vi "2022_day12.vi"() -> ()   [LabVIEW 2021]
uses:
  <vilib>/Utility/miscctls.llb/LVRowAndColumnTypeDef.ctl
panel:
  out "Table Control":string[][](table)
  out "Array":string[][](array[string])
  out "Searching progress":i32[][](array[numeric])
  out "Input Data":i32[][](array[numeric])
  out "Task 1":i32
  in  "Switch":bool caption="Ex. Data  vs.  User Data"
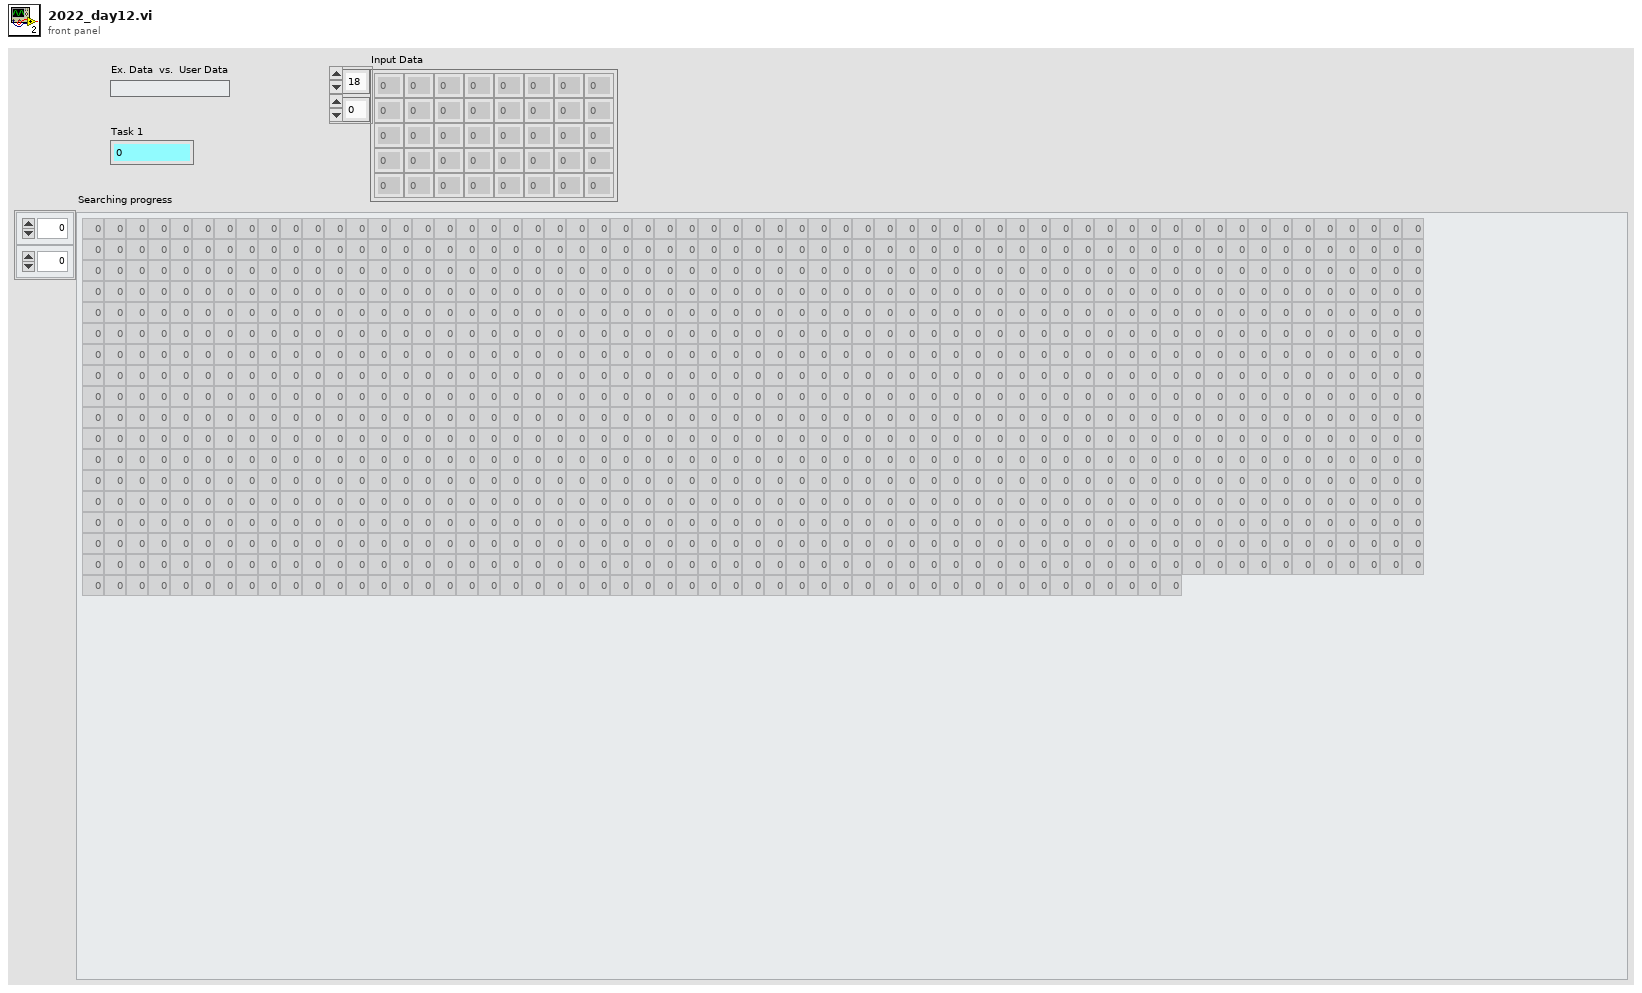
[diagram p1: front panel]
types:
  T1 = typedef "LVRowAndColumnTypeDef.ctl" = cluster{"Row":i32, "Column":i32}
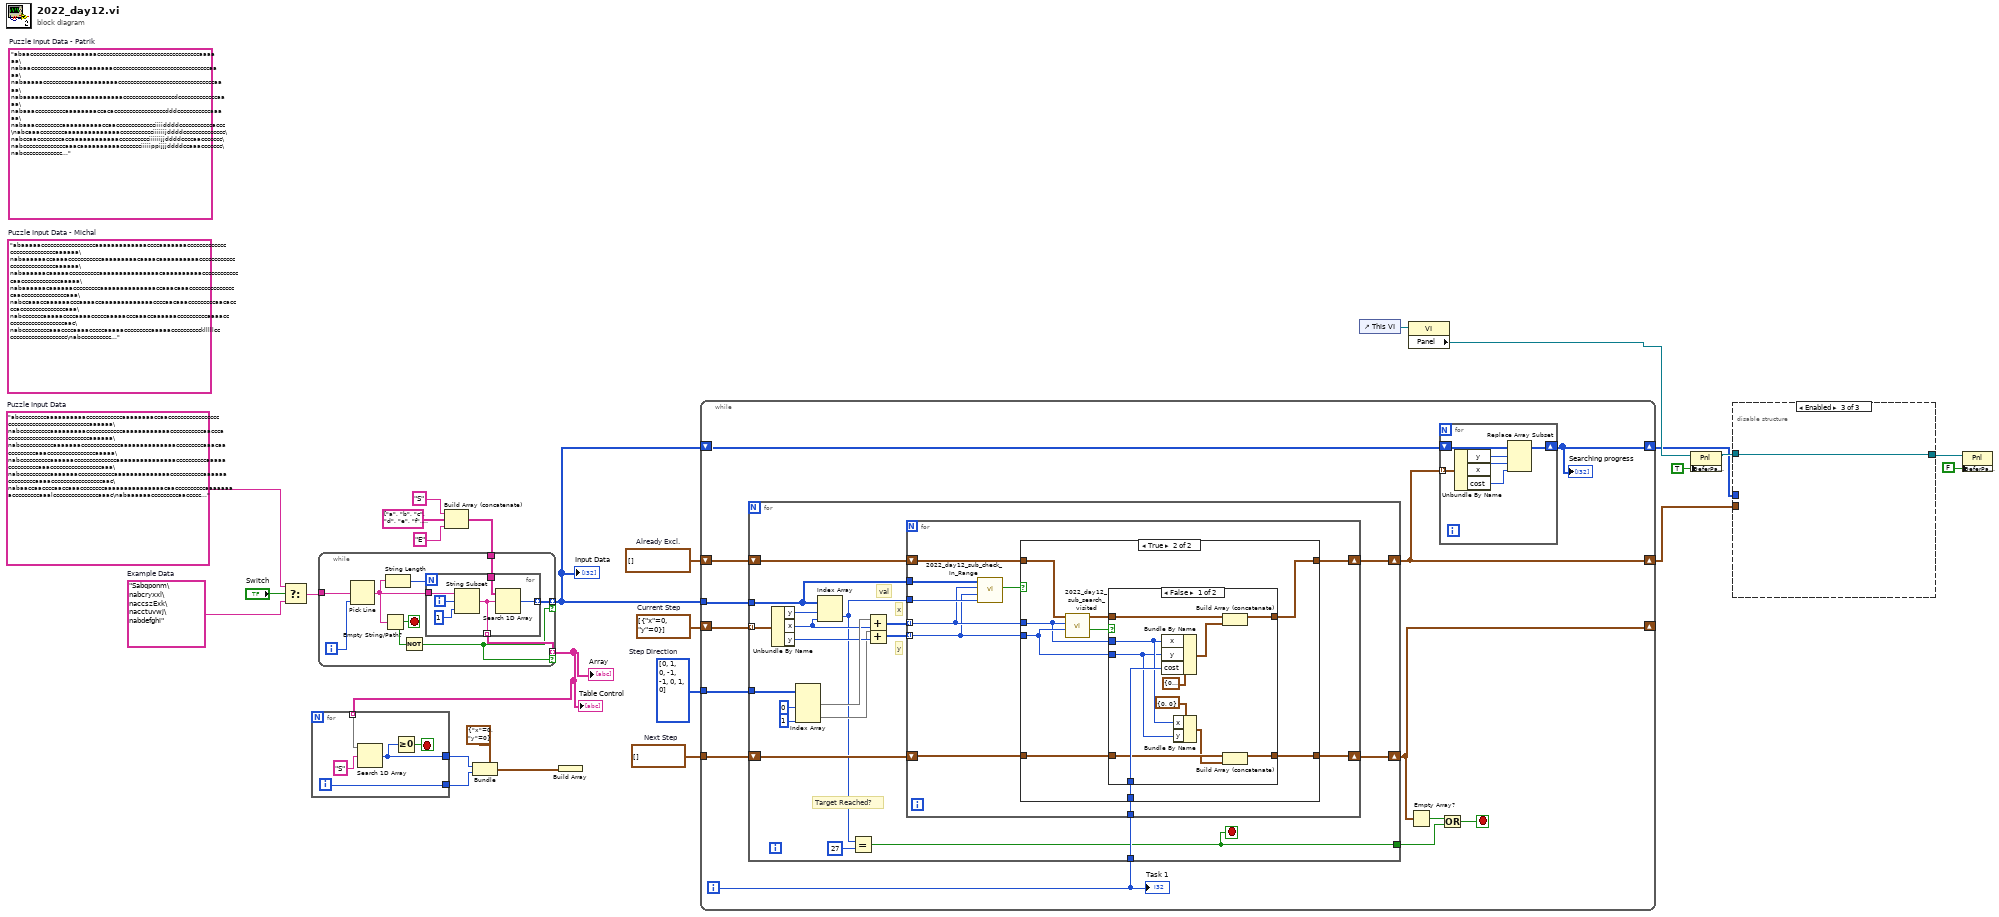
[diagram p0: block diagram]
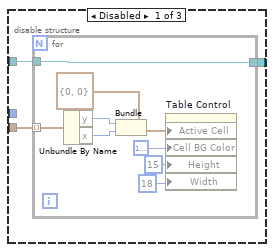
[diagram p2: hidden frame]
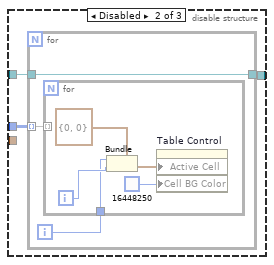
[diagram p3: hidden frame]
diagram:
  (unwired) "abaacccccccccccccaaaaaaaccccccccccccccccccccccccccccccccccaaaaaa\nabaaccccccccccccccaaaaaaaaaaccccccccccccccccccccccccccccccccaaaa\nabaaaaacccccccccaaaaaaaaaaaaccccccccccccccccccccccccccccccccaaaa\nabaaaaaccccccccaaaaaaaaaaaaaacccccccccccccccccdcccccccccccccaaaa\nabaaaccccccccccaaaaaaaaccacacccccccccccccccccdddcccccccccccaaaaa\nabaaacccccccccaaaaaaaaaaccaaccccccccccccciiiiddddcccccccccccaccc\nabcaaaccccccccaaaaaaaaaaaaaaccccccccccciiiiiijddddcccccccccccccc\nabccaaccccccccaccaaaaaaaaaaaacccccccccciiiiiijjddddccccaaccccccc\nabccccccccccccccaaacaaaaaaaaaaccccccciiiiippijjjddddccaaaccccccc\nabccccccccccccc..."  # Puzzle Input Data - Patrik
  (unwired) "abaaaaaccccccccccccccccccaaaaaaaaaaaaaccccaaaaaaaccccccccccccccccccccccccccccaaaaaa\nabaaaaaaccaaaacccccccccccaaaaaaaaacaaaacaaaaaaaaaacccccccccccccccccccccccccccaaaaaa\nabaaaaaacaaaaaccccccccccaaaaaaaaaaaaaaacaaaaaaaaaacccccccccccccaacccccccccccccaaaaa\nabaaaaaacaaaaaacccccccccaaaaaaaaaaaaaaccaaacaaaccccccccccccccccaacccccccccccccccaaa\nabccaaaccaaaaaacccaaaaccaaaaaaaaaaaaaccccaacaaacccccccccaacaccccacccccccccccccccaaa\nabcccccccaaaaaccccaaaacccccaaaaacccaaaccaaaaaaccccccccccaaaaccccccccccccccccccccaac\nabcccccccccaaaccccaaaacccccaaaaacccccccccaaaaaccccccccccklllllccccccccccccccccccccc\nabcccccccccc..."  # Puzzle Input Data - Michal
  w17 = cluster{"x":i32, "y":i32}[] []  # Next Step
  w2 = cluster{"x":i32, "y":i32}[] [{"x"=0, "y"=0}]  # Current Step
  w18 = i32[][] [[0, 1], [0, -1], [-1, 0], [1, 0]]  # Step Direction
  w19 = cluster{"x":i32, "y":i32, "cost":i32}[] []  # Already Excl.
  w1 = "abcccccccccaaaaaaaaaaccccccccccccaaaaaaaaccaaccccccccccccccccccccccccccccccccccccccccccccaaaaaa\nabccccccccccaaaaaaaaaccccccccccccaaaaaaaaaaaacccccccccccaacccacccccccccccccccccccccccccccaaaaaa\nabcccccccccccaaaaaaacccccccccccccaaaaaaaaaaaaaacccccccccaaacaacccccccccaaaccccccccccccccccaaaaa\nabccccccccccaaaaaaccccccccccccccaaaaaaaaaaaaaaaccccccccccaaaaaccccccccccaaacccccccccccccccccaaa\nabccccccccccaaaaaaaccccccccccccaaaaaaaaaaaaaacccccccccccaaaaaacccccccccaaaacccccccccccccccccaac\nabaaccaaccccaaccaaaccccccccaaaaaaaaaaaaaaacaaccccccccccaaaaaaaacccccccccaaalcccccccccccccccaaac\nabaaaaaacccccccccaaccccc..."  # Puzzle Input Data
  w25 = "Sabqponm\nabcryxxl\naccszExk\nacctuvwj\nabdefghi"  # Example Data
  n1 = Select(t=w1, s="Switch", f=w25) -> (s? t:f=w24:string)
  n2 = Build Array (concatenate)("S" ("format string"), string[] ["a", "b", "c", "d", "e", "f", "g", "h", "i", "j", "k", "l", "m", "n", "o", "p", "q", "r", "s", "t", "u", "v", "w", "x", "y", "z"] ("all lower case string"), "E" ("format string")) -> (w20:string[])
  n3 = while {
    tunnel: w24 -> [w35]
    tunnel: [w31] -> w16 mode=indexing if=w27
    tunnel: w20 -> [w29]
    tunnel: [w28] -> w14 mode=indexing if=w27
    i -> [w34]
    stop <- w30 stop-if-true
    n4 = Pick Line(multi-line string=w35, line index=w34) -> (output string=w32:string)  [unwired: 1 in]
    n5 = Empty String/Path?(string/path=w32) -> (empty?=w30:bool)
    n6 = String Length(string=w32) -> (length=w33:i32)
    n7 = Not(x=w30) -> (.not. x?=w27:bool)
    n8 = for {
      N: w33 -> [_]
      tunnel: [w38] -> w31 mode=indexing
      tunnel: w32 -> [w39]
      tunnel: w29 -> [w37]
      tunnel: [w36] -> w28 mode=indexing
      i -> [w41]
      n9 = String Subset(string=w39, offset (0)=w41, length (rest)=1 ("length (rest)")) -> (substring=w36:string)
      n10 = Search 1D Array(1D array=w37, element=w36) -> (index of element=w38:i32)  [unwired: 1 in]
    }
  }
  "Input Data" <- w16
  "Array" <- w14
  "Table Control" <- w14
  n11 = for {
    tunnel: w14 -> [w46] mode=indexing
    tunnel: [w43] -> w11
    tunnel: [w42] -> w10
    i -> [w43]
    stop <- w44 stop-if-true
    n12 = Search 1D Array(1D array=w46, element="S" ("format string")) -> (index of element=w42:i32)  [unwired: 1 in]
    n13 = Greater Or Equal To 0?(x=w42) -> (x >= 0?=w44:bool)
  }
  n14 = Bundle(cluster=cluster{"x":i32, "y":i32} {"x"=0, "y"=0} ("point"), "x"=w10, "y"=w11) -> (w12:cluster{"x":i32, "y":i32})
  n15 = Build Array(w12) -> ()  [unwired: 1 out]
  n16 = while {
    tunnel: w16 -> [w59]
    shift-right: [w49] -> w5
    shift-left: w19 -> [w57]
    shift-right: [w47] -> _
    shift-left: w2 -> [w56]
    tunnel: w18 -> [w58]
    tunnel: w17 -> [w55]
    shift-right: [w53] -> w3
    shift-left: w16 -> [w54]
    i -> [w48]
    stop <- w51 stop-if-true
    n17 = for {
      tunnel: w56 -> [w84] mode=indexing
      tunnel: w59 -> [w73]
      tunnel: w58 -> [w83]
      shift-right: [w72] -> w49
      shift-left: w57 -> [w74]
      shift-right: [w70] -> w47
      shift-left: w55 -> [w71]
      tunnel: w48 -> [w69]
      tunnel: [w66] -> w52
      stop <- w66 stop-if-true
      # "Target Reached?"
      # "val"
      # "y"
      # "x"
      n18 = Unbundle By Name(w84) -> ("y"=w85:i32, "x"=w79:i32, "y"=w78:i32)
      n19 = Index Array(array=w83, index (col) #1=0 ("disabled index (col)"), index (col) #2=1 ("index (col)")) -> (element #1=w80:i32[], element #2=w75:i32[])  [unwired: 2 in]
      n20 = Index Array(array=w73, index (row)=w85, index (col)=w79) -> (element=w67:i32)
      n21 = Equal?(x=w67, y=27) -> (x = y?=w66:bool)
      n22 = Add(x=w80, y=w79) -> (x+y=w77:i32[])
      n23 = Add(x=w75, y=w78) -> (x+y=w76:i32[])
      n24 = for {
        tunnel: w77 -> [w91] mode=indexing
        tunnel: w76 -> [w90] mode=indexing
        tunnel: w67 -> [w92]
        tunnel: w73 -> [w93]
        shift-right: [w88] -> w72
        shift-left: w74 -> [w95]
        tunnel: w69 -> [w89]
        shift-right: [w87] -> w70
        shift-left: w71 -> [w86]
        n25 = call "2022_day12_sub_check_In_Range.vi"("Val Current"=w92, "Y"=w90, "X"=w91, "Playboard"=w93) -> ("Checkbox"=w94:bool)  [unwired: 7 in]
        n26 = case shown="True" w94 {
          tunnel: w95 -> [w97 w106]
          tunnel: w90 -> [_ w104]
          tunnel: w91 -> [_ w103]
          tunnel: w89 -> [_ w105]
          tunnel: [w97 w101] -> w88
          tunnel: [w96 w99] -> w87
          tunnel: w86 -> [w96 w100]
          frame False {
          }
          frame True {
            n27 = call "2022_day12_sub_search_visited.vi"("Val Y"=w104, "Val X"=w103, "Already Excl In."=w106) -> ("Point Found?"=w98:bool, "Already Excl. Out"=w102:cluster{"x":i32, "y":i32, "cost":i32}[])  [unwired: 7 in]
            n28 = case shown="False" w98 {
              tunnel: w105 -> [w116 _]
              tunnel: w104 -> [w107 _]
              tunnel: w103 -> [w108 _]
              tunnel: w102 -> [w115 w119]
              tunnel: [w114 w119] -> w101
              tunnel: w100 -> [w112 w118]
              tunnel: [w111 w118] -> w99
              frame False {
                n29 = Bundle By Name(cluster=cluster{"x":i32, "y":i32, "cost":i32} {"x"=0, "y"=0, "cost"=0} ("point"), "x"=w108, "y"=w107, "cost"=w116) -> (w113:cluster{"x":i32, "y":i32, "cost":i32})
                n30 = Bundle By Name(cluster=cluster{"x":i32, "y":i32} {"x"=0, "y"=0} ("point"), "x"=w108, "y"=w107) -> (w109:cluster{"x":i32, "y":i32})
                n31 = Build Array (concatenate)(w115, w113) -> (w114:cluster{"x":i32, "y":i32, "cost":i32}[])
                n32 = Build Array (concatenate)(w112, w109) -> (w111:cluster{"x":i32, "y":i32}[])
              }
              frame True {
              }
            }
          }
        }
      }
    }
    n33 = Empty Array?(array=w47) -> (empty?=w50:bool)
    n34 = for {
      shift-right: [w61] -> w53
      shift-left: w54 -> [w64]
      tunnel: w49 -> [w65] mode=indexing
      n35 = Unbundle By Name(w65) -> ("y"=w63:i32, "x"=w62:i32, "cost"=w60:i32)
      n36 = Replace Array Subset(array=w64, new element=w60, index (row)=w63, index (col)=w62) -> (w61:i32[][])
    }
    "Searching progress" <- w53
    n37 = Or(x=w50, y=w52) -> (x .or. y?=w51:bool)
    "Task 1" <- w48
  }
  n38 = control-ref of="This VI"() -> (w15:refnum<vi>)
  n39 = property class="VI"(reference=w15) -> ("Panel"=w4:refnum<vi>)  [unwired: 1 in, 2 out]
  n40 = property class="Pnl"(reference=w4, "DeferPanUpdts"=TRUE ("Defer Panel Updates")) -> (reference out=w8:refnum<vi>)  [unwired: 1 in, 1 out]
  n41 = disable-structure shown="Enabled" {
    disable-tunnel: [w122 w133 w143] -> w9
    disable-tunnel: w8 -> [w121 w134 w143]
    disable-tunnel: w3 -> [_ w132 _]
    disable-tunnel: w5 -> [w120 _ _]
    frame Disabled {
      n42 = for {
        tunnel: [w126] -> w122
        tunnel: w121 -> [w126]
        tunnel: w120 -> [w123] mode=indexing
        n43 = Unbundle By Name(w123) -> ("y"=w129:i32, "x"=w128:i32)
        n44 = Bundle(cluster=T1 {"Row"=0, "Column"=0} ("Active Cell:Active Cell"), "Row"=w129, "Column"=w128) -> (w130:T1)
        n45 = property on="Table Control" class="Tbl (strict)"("Active Cell"=w130, "Cell BG Color"=u32 16777226, "Height"=u32 15 ("Active Cell:Cell Size:Height"), "Width"=u32 18 ("Active Cell:Cell Size:Width")) -> ()  [unwired: 2 in, 2 out]
      }
    }
    frame Disabled {
      n46 = for {
        tunnel: w134 -> [w136]
        tunnel: [w136] -> w133
        tunnel: w132 -> [w135] mode=indexing
        i -> [w137]
        n47 = for {
          tunnel: w137 -> [w138]
          tunnel: w135 -> [_] mode=indexing
          i -> [w139]
          n48 = Bundle(cluster=T1 {"Row"=0, "Column"=0} ("Active Cell:Active Cell"), "Row"=w138, "Column"=w139) -> (w142:T1)
          n49 = property on="Table Control" class="Tbl (strict)"("Active Cell"=w142, "Cell BG Color"=u32 16448250) -> ()  [unwired: 2 in, 2 out]
        }
      }
    }
    frame Enabled {
    }
  }
  n50 = property class="Pnl"(reference=w9, "DeferPanUpdts"=FALSE ("Defer Panel Updates")) -> ()  [unwired: 1 in, 2 out]
